vi "Source Current V3.vi"(8 "error in":errorcluster, 10 "Current Level (A)":dbl format="%#_6p", 11 "DCPower SSC in":T1[](array[typedef])) -> (0 "error out":errorcluster, 3 "DCPower SSC out":T1[](array[typedef]))   [LabVIEW 2019]
uses:
  Instrument Control/DCPower/SSC DCPower/SSC DCPower.ctl
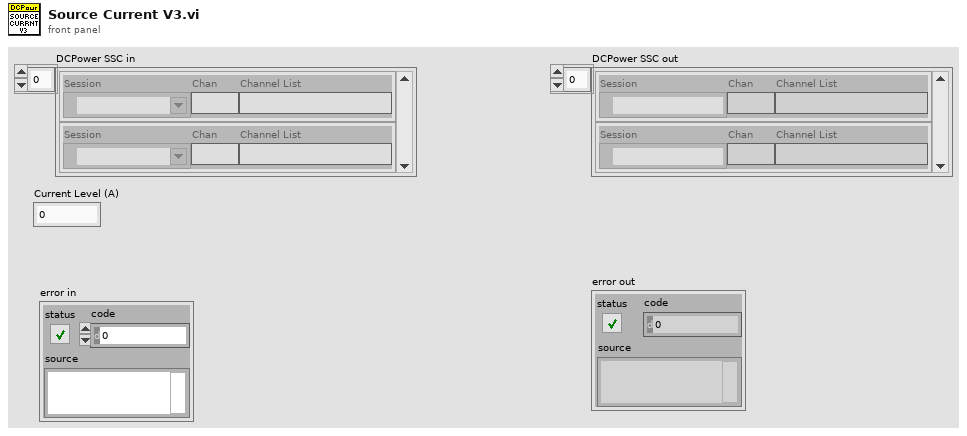
[diagram p1: front panel]
types:
  T1 = typedef "SSC DCPower.ctl" = cluster{"Session":refnum<k15>, "Chan":string, "Channel List":string}
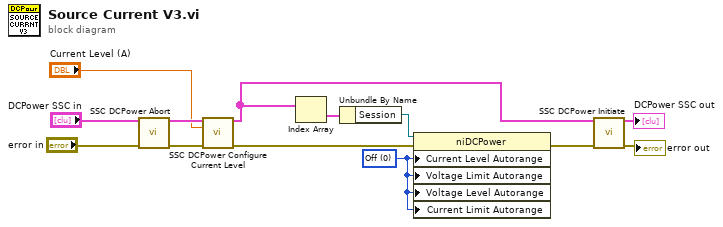
[diagram p0: block diagram]
diagram:
  w4 = 0 items=["Off", "On"] ("Source:DC Voltage:Voltage Level Autorange")
  n1 = call "SSC DCPower Abort.vi"("DCPower SSC in"="DCPower SSC in", "error in"="error in") -> ("DCPower SSC out"=w9:T1[], "error out"=w8:errorcluster)  [unwired: 12 in]
  n2 = call "SSC DCPower Configure Current Level.vi"("DCPower SSC in"=w9, "Current Level (A)"="Current Level (A)", "error in"=w8) -> ("DCPower SSC out"=w1:T1[], "error out"=w3:errorcluster)  [unwired: 11 in]
  n3 = Index Array(array=w1) -> (element=w6:T1)  [unwired: 1 in]
  n4 = Unbundle By Name(w6) -> ("Session"=w5:refnum<k15>)
  n5 = property class="niDCPower"(reference=w5, error in=w3, "Current Level Autorange"=w4, "Voltage Limit Autorange"=w4, "Voltage Level Autorange"=w4, "Current Limit Autorange"=w4) -> (error out=w2:errorcluster)  [unwired: 1 out]
  n6 = call "SSC DCPower Initiate.vi"("DCPower SSC in"=w1, "error in"=w2) -> ("DCPower SSC out"=→"DCPower SSC out":T1[], "error out"=→"error out":errorcluster)  [unwired: 12 in]
